vi "CurrentCellDirtyStateChanged Event Callback.vi"(4 "DataGridView in":refnum<class "DataGridView.lvclass">, 5 "Event Data":cluster{"sender":refnum<k24>, "e":refnum<k24>}, 6 "Control Ref":refnum<k24>, 7 "Event Common Data":T1) -> ()   [LabVIEW 2013, in "DataGrid.lvlib" / "DataGridView.lvclass"]
doc: "The CurrentCellDirtyStatChanged event is triggered when a checkbok or combo box has changed state but focus has not moved to another location in the DataGridView. This callback commits the change and will then trigger a ValueChanged event."
uses:
  DataGridView/DataGridView.lvclass
  System.Windows.Forms
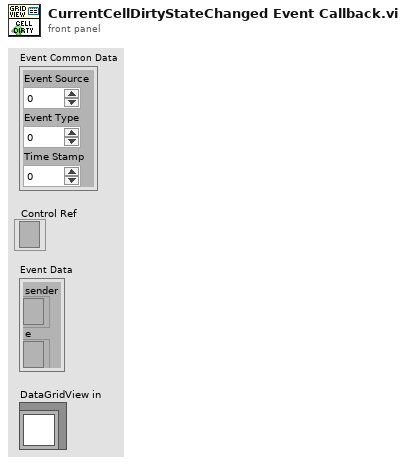
[diagram p1: front panel]
types:
  T1 = cluster{"Event Source":i32, "Event Type":u32, "Time Stamp":u32}
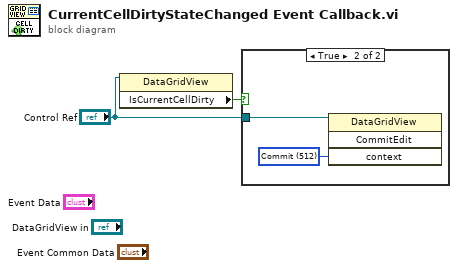
[diagram p0: block diagram]
diagram:
  n1 = property class="DataGridView"(reference="Control Ref") -> ("IsCurrentCellDirty"=w1:bool)  [unwired: 1 in, 2 out]
  n2 = case shown="True" w1 {
    tunnel: "Control Ref" -> [_ w4]
    frame False {
    }
    frame True {
      w3 = 512 items=["Formatting"=1, "Display"=2, "PreferredSize"=4, "RowDeletion"=8, "Parsing"=256, "Commit"=512, "InitialValueRestoration"=1024, "LeaveControl"=2048, "CurrentCellChange"=4096, "Scroll"=8192, "ClipboardContent"=16384] ("context")
      n3 = invoke class="DataGridView" method="CommitEdit"(reference=w4, "context"=w3) -> ()  [unwired: 2 in, 4 out]
    }
  }
